vi "Init.vi"(0 "Gen2 in":refnum<class "KDemoDerived.lvclass">, 7 "Variant":variant, 9 "Prefix":string="Derived", 11 "error in (no error)":errorcluster) -> (4 "Gen2 out":refnum<class "KDemoDerived.lvclass">, 15 "error out":errorcluster)   [LabVIEW 2015, in "KDemoDerived.lvclass"]
uses:
  KDemoDerived.lvclass
  KDemoDerived.lvclass/KDemoDerived.ctl
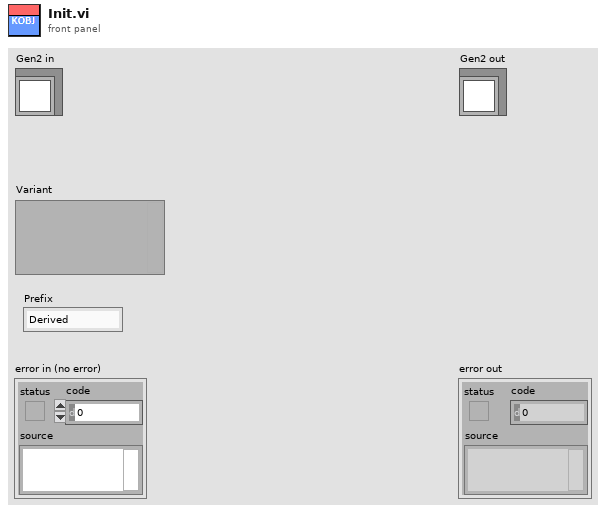
[diagram p1: front panel]
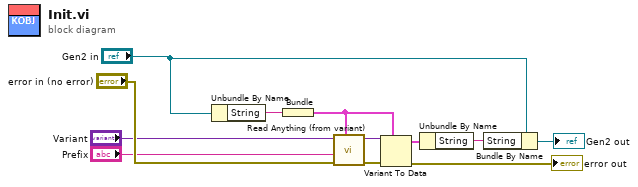
[diagram p0: block diagram]
diagram:
  n1 = Unbundle By Name("Gen2 in") -> ("String"=w10:string)
  n2 = Bundle("String"=w10) -> (w7:cluster{"String":string})  [unwired: 1 in]
  n3 = call "Read Anything (from variant).vi"("Type of Anything"=w7, "Error In"="error in (no error)", "Prefix"="Prefix", "Variant Database"="Variant") -> ("Error Out"=w9:errorcluster, "Anything"=w8:variant)  [unwired: 5 in, 1 out]
  n4 = Variant To Data(error in=w9, type=w7, Variant=w8) -> (data=w6:cluster{"String":string}, error out=→"error out":errorcluster)
  n5 = Unbundle By Name(w6) -> ("String"=w5:string)
  n6 = Bundle By Name(cluster="Gen2 in", "String"=w5) -> (→"Gen2 out":refnum<class "KDemoDerived.lvclass">)
